vi "Get area size.vi"(8 "error in (no error)":errorcluster, 10 "Sub Panel":refnum<vi>, 11 "DualScreenH in":refnum<class "DualScreenH.lvclass">) -> (0 "error out":errorcluster, 2 "Area size (px)":u32, 3 "DualScreenH out":refnum<class "DualScreenH.lvclass">)   [LabVIEW 2020, in "DualScreenH.lvlib" / "DualScreenH.lvclass"]
uses:
  DualScreenH.lvclass
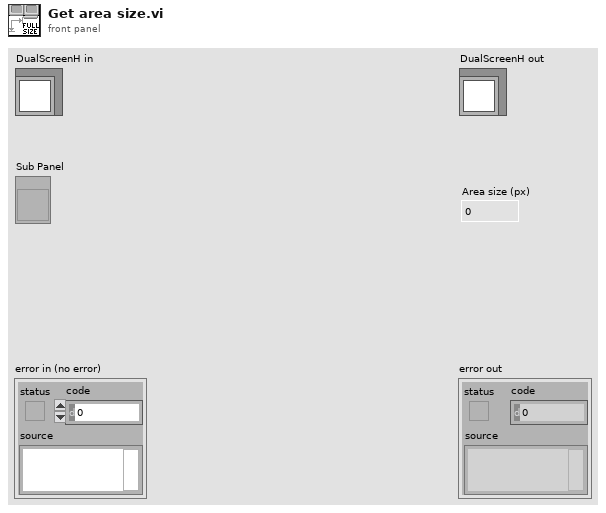
[diagram p1: front panel]
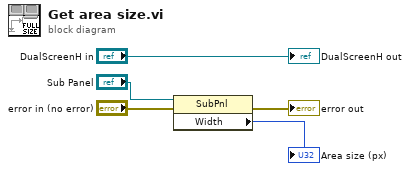
[diagram p0: block diagram]
diagram:
  n1 = property class="SubPnl"(reference="Sub Panel", error in="error in (no error)") -> (error out=→"error out":errorcluster, "Width"=→"Area size (px)":u32)  [unwired: 1 out]
  "DualScreenH out" <- "DualScreenH in"
